vi "Behaviour Tree.vi"(8 "error in (no error)":errorcluster, 11 "IO":T1) -> (0 "error out":errorcluster, 2 "Behaviour Tree":refnum<class "bt_Node.lvclass">)   [LabVIEW 2021]
uses:
  Support/IO_Type.ctl
  <vilib>/TSA/Event Log/Event_TextLog/Event_TextLog.lvclass
  C:/Program Files (x86)/National Instruments/LabVIEW 2021/vi.lib/TSA/Event Log/abs_EventLog/abs_EventLog.lvclass
  Blackboard/Blackboard.lvclass
  Support/Nodes/abs_Node/bt_Node.lvclass
  Support/Nodes/Leaves/Log/bt_Log.lvclass
  C:/Users/timst/Documents/Repositories/LV_Behaviour_Tree/Source/Support/Nodes/abs_Node/bt_Node.lvclass
  Support/Poly/Log/Log_String.vi
  BT.lvlib
  C:/Program Files (x86)/National Instruments/LabVIEW 2021/vi.lib/TSA/Event Log/Event_TextLog/Event_TextLog.lvclass
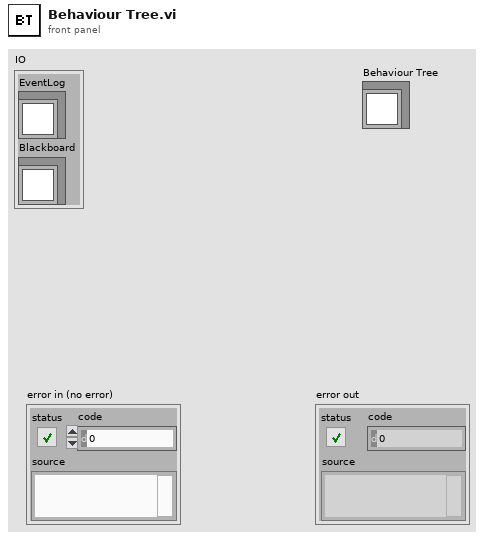
[diagram p1: front panel]
types:
  T1 = typedef "IO_Type.ctl" = cluster{"EventLog":refnum<class "Event_TextLog.lvclass">, "Blackboard":refnum<class "Blackboard.lvclass">}
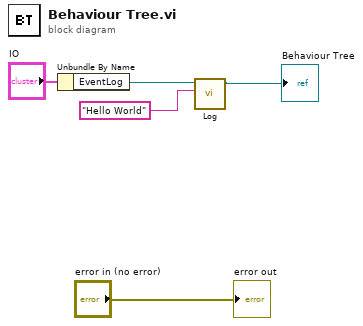
[diagram p0: block diagram]
diagram:
  n1 = Unbundle By Name("IO") -> ("EventLog"=w2:refnum<class "Event_TextLog.lvclass">)
  n2 = call-poly "Log.vi"("Message"="Hello World", "EventLog"=w2) -> ("node out"=→"Behaviour Tree":refnum<class "bt_Log.lvclass">)  [unwired: 9 in]
  "error out" <- "error in (no error)"
